vi "RegisterReaderSockets.vi"(7 "error in (no error)":errorcluster, 8 "IP":string="172.16.7.43", 10 "Port":u16=9764) -> (0 "error out":errorcluster)   [LabVIEW 2009]
panel:
  in  "Register Number":u16=4
  out "Register Read":dbl[](array[numeric])
  out "Register read":u32
  in  "Device":u16(ring)=4 items=["Attenuation", "Clipping", "Enable channel", "Delay line", "ASIC"]
  # "0     1     2     3     4    5     6     7     8    9    10   11  12   13   14   15"
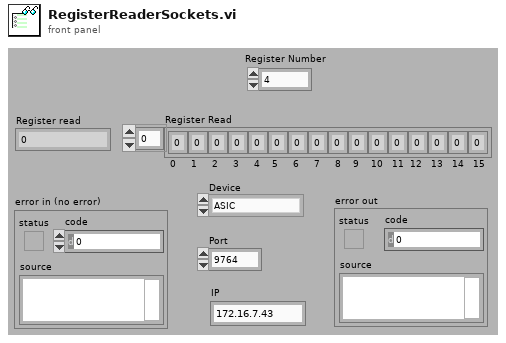
[diagram p1: front panel]
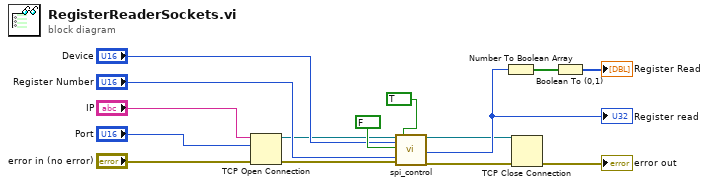
[diagram p0: block diagram]
diagram:
  n1 = TCP Open Connection(address="IP", remote port or service name="Port", error in (no error)="error in (no error)") -> (connection ID=w7:refnum<k5>, error out=w5:errorcluster)  [unwired: 2 in]
  n2 = call "spi_control.vi"("connection ID"=w7, "Device"="Device", "Read/#write"=FALSE, "Register or channel"="Register Number", "error out 3"=w5, "Read physical"=TRUE) -> ("connection ID out"=w2:refnum<k5>, "data read value"=w12:u32, "error out 2"=w4:errorcluster)  [unwired: 6 in, 5 out]
  "Register read" <- w12
  n3 = Number To Boolean Array(number=w12) -> (Boolean array=w14:bool[])
  n4 = TCP Close Connection(connection ID=w2, error in (no error)=w4) -> (error out=→"error out":errorcluster)  [unwired: 1 in, 1 out]
  n5 = Boolean To (0,1)(Boolean=w14) -> (0, 1=→"Register Read":i16[])
